vi "SaveSpectrometerData.vi"(7 "Average":dbl, 8 "error in (no error)":errorcluster, 9 "Wavelengths":dbl[](array[numeric]), 10 "Color Temperatures":dbl[][](array[numeric]), 11 "Refnum in":refnum<k34>) -> (0 "error out":errorcluster, 3 "Refnum out":refnum<k34>)   [LabVIEW 2018]
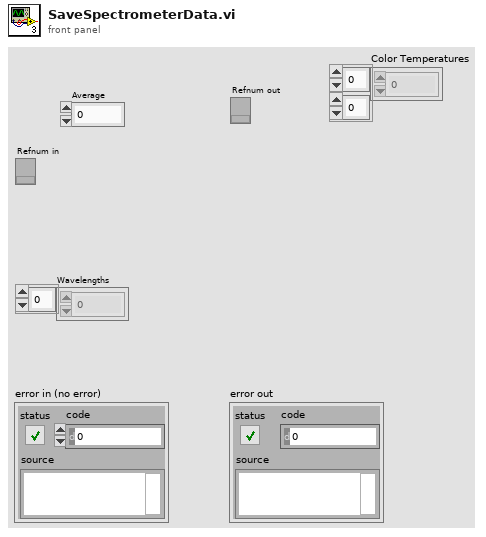
[diagram p1: front panel]
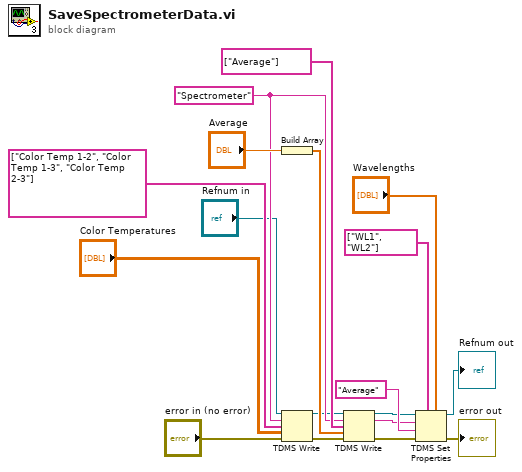
[diagram p0: block diagram]
diagram:
  w7 = "Spectrometer" ("group name in (Untitled)")
  n1 = Build Array("Average") -> (w8:dbl[])
  n2 = TDMS Write(0:"Refnum in", 5:w7, 7:string[] ["Color Temp 1-2", "Color Temp 1-3", "Color Temp 2-3"] ("channel name(s) in (Untitled)"), 9:"Color Temperatures", 11:"error in (no error)") -> (4:w2:refnum<k34>, 15:w1:errorcluster)  [unwired: 1 in, 2 out]
  n3 = TDMS Write(0:w2, 5:w7, 7:string[] ["Average"] ("channel name(s) in (Untitled)"), 9:w8, 11:w1) -> (4:w15:refnum<k34>, 6:w14:string, 15:w13:errorcluster)  [unwired: 1 in, 1 out]
  n4 = TDMS Set Properties(5:"Wavelengths", 7:string[] ["WL1", "WL2"] ("property names"), 8:w13, 9:"Average", 10:w14, 11:w15) -> (0:→"error out":errorcluster, 3:→"Refnum out":refnum<k34>)  [unwired: 2 out]
